vi "LJM_INT32ToByteArray.vi"(1 "I32":i32) -> (0 "Byte Array":u8[](array[numeric]))   [LabVIEW 2020]
panel:
  # "Converts a I32 to a 4-element big-endian byte array."
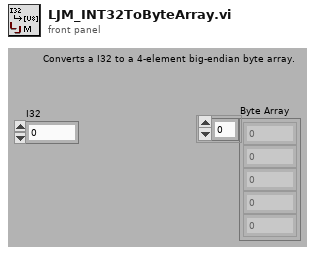
[diagram p1: front panel]
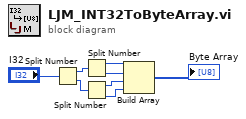
[diagram p0: block diagram]
diagram:
  n1 = Split Number(x="I32") -> (hi(x)=w6:u16, lo(x)=w5:u16)
  n2 = Split Number(x=w6) -> (hi(x)=w4:u8, lo(x)=w3:u8)
  n3 = Split Number(x=w5) -> (hi(x)=w2:u8, lo(x)=w1:u8)
  n4 = Build Array(w4, w3, w2, w1) -> (→"Byte Array":u8[])
